vi "splitAudioStreamsIntoSeparateTracks.vi"(8 "error in (no error)":errorcluster, 10 "Number of streams":i32, 11 "Audio path":path) -> (0 "error out":errorcluster, 1 "return code":i32)   [LabVIEW 2017]
doc: "Invoke ffmpeg to combine audio and video files into a single .avi file.\n\nRequires that ffmpeg be installed on the system."
panel:
  out "resulting string":string
  out "Post system call error":errorcluster
  out "standard output":string
  out "standard error":string
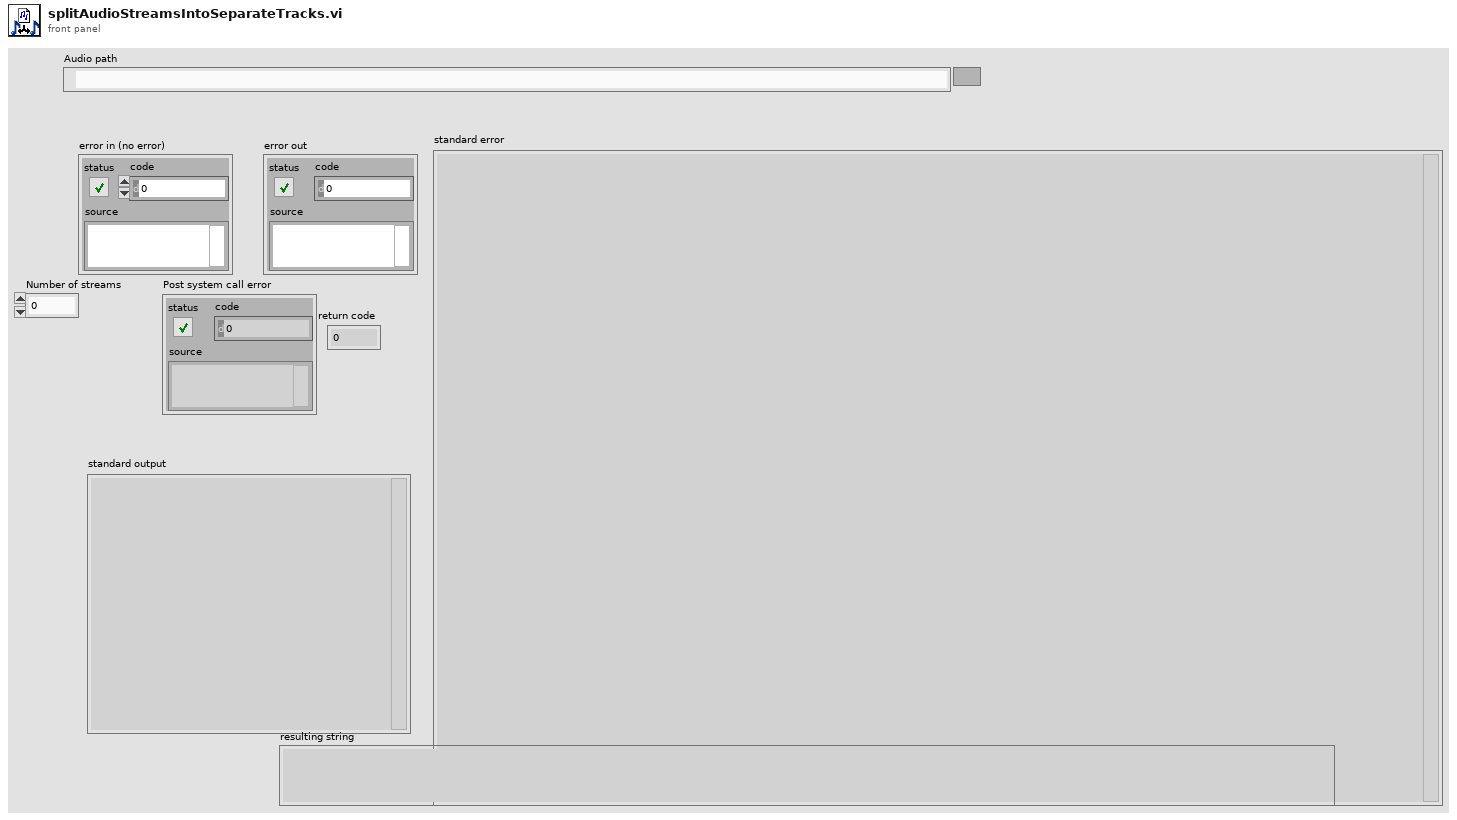
[diagram p1: front panel]
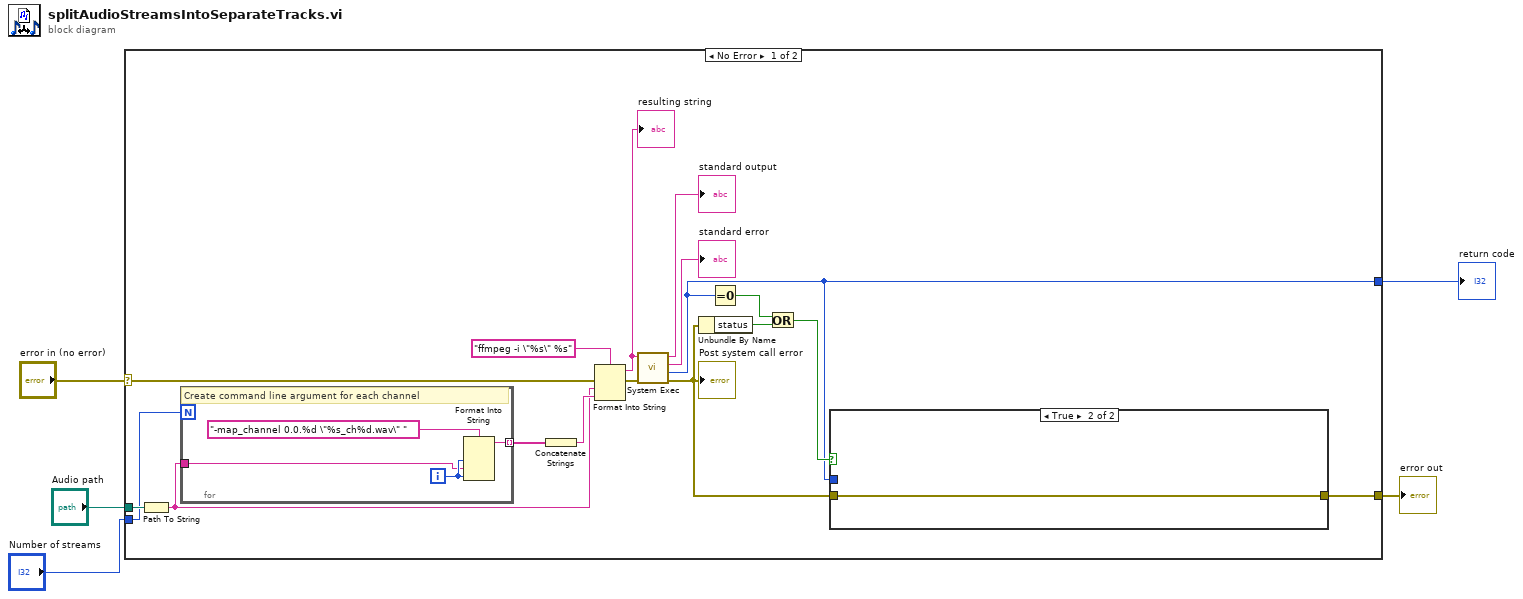
[diagram p0: block diagram]
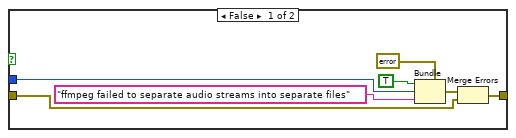
[diagram p2: hidden frame]
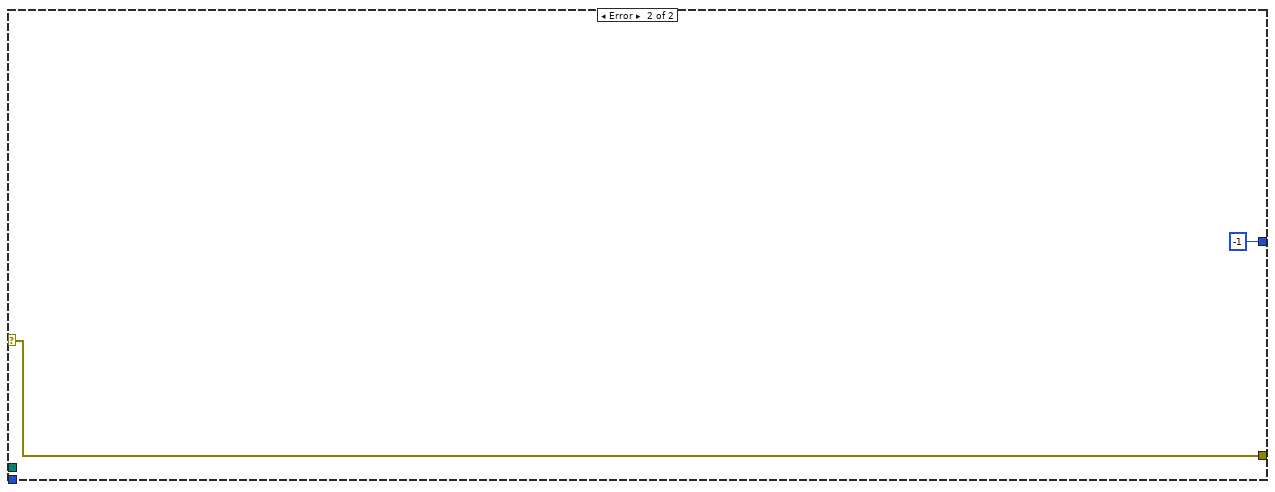
[diagram p3: hidden frame]
diagram:
  n1 = case shown="No Error" "error in (no error)" {
    selector: "error in (no error)" -> [w14 w36]
    tunnel: [w13 w36] -> w4
    tunnel: "Audio path" -> [w11 _]
    tunnel: [w10 -1 ("return code")] -> w2
    tunnel: "Number of streams" -> [w9 _]
    frame No Error {
      n2 = Path To String(path=w11) -> (string=w6:string)
      n3 = for {
        N: w9 -> [_]
        tunnel: [w25] -> w8 mode=indexing
        tunnel: w6 -> [w23]
        i -> [w24]
        # "Create command line argument for each channel"
        n4 = Format Into String(format string="-map_channel 0.0.%d \"%s_ch%d.wav\" " ("command line"), w24, w23, w24) -> (resulting string=w25:string)  [unwired: 2 in, 1 out]
      }
      n5 = Concatenate Strings(w8) -> (w7:string)
      n6 = Format Into String(format string="ffmpeg -i \"%s\" %s" ("command line"), error in=w14, w6, w7) -> (resulting string=w22:string, error out=w21:errorcluster)  [unwired: 1 in]
      "resulting string" <- w22
      n7 = call <vilib>:"System Exec.vi"("error in (no error)"=w21, "command line"=w22) -> ("error out"=w17:errorcluster, "return code"=w10:i32, "standard error"=→"standard error":string, "standard output"=→"standard output":string)  [unwired: 6 in]
      "Post system call error" <- w17
      n8 = Unbundle By Name(w17) -> ("status"=w15:bool)
      n9 = Equal To 0?(x=w10) -> (x = 0?=w12:bool)
      n10 = Or(x=w12, y=w15) -> (x .or. y?=w16:bool)
      n11 = case shown="True" w16 {
        tunnel: w17 -> [w27 w34]
        tunnel: [w28 w34] -> w13
        tunnel: w10 -> [w31 _]
        frame False {
          n12 = Bundle(cluster=errorcluster {"status"=FALSE, "code"=0, "source"=""} ("error out"), "status"=TRUE, "code"=w31, "source"="ffmpeg failed to separate audio streams into separate files") -> (w33:errorcluster)
          n13 = Merge Errors(w33, w27) -> (w28:errorcluster)
        }
        frame True {
        }
      }
    }
    frame Error {
    }
  }
  "error out" <- w4
  "return code" <- w2
